vi "Initialize Sweep Waveform.vi"(8 "error in (no error)":errorcluster, 11 "Instrument.DAQ in":refnum<class "Instrument.DAQ.lvclass">) -> (0 "error out":errorcluster, 2 "Waveforms":waveform(dbl)[](array[waveform]), 3 "Instrument.DAQ out":refnum<class "Instrument.DAQ.lvclass">)   [LabVIEW 2019, in "Instrument.Lockin.lvlib" / "Instrument.DAQ.lvclass"]
uses:
  Instrument.DAQ.lvclass
  Instrument.DAQ.lvclass/Instrument.DAQ.ctl
  <vilib>/Utility/error.llb/Error Cluster From Error Code.vi
  <vilib>/ErrorRing/Error Ring.xnode
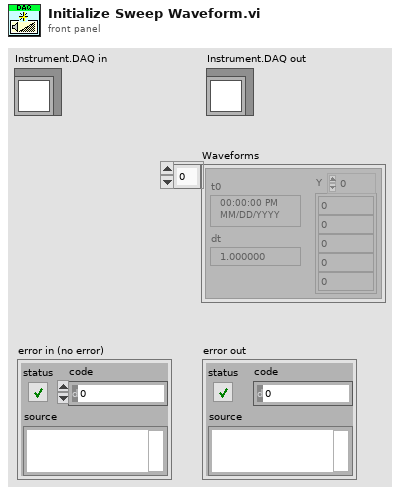
[diagram p1: front panel]
types:
  T1 = typedef "Instrument.Lockin.lvlib/Instrument.DAQ.lvclass/AO.Channel--Cluster--Array.ctl" = T2[]
  T2 = typedef "Instrument.Lockin.lvlib/Instrument.DAQ.lvclass/AO.Channel--Cluster.ctl" = cluster{"Enable?":bool, "Channel":i32, "Amplitude":dbl, "Offset":dbl, "Frequency":dbl, "Phase":dbl, "Function":T3, "Sweeping?":bool}
  T3 = typedef "Instrument.Lockin.lvlib/Instrument.DAQ.lvclass/AO.Channel.Function--Enum.ctl" = enum16{"Sine", "Triangle", "Square"}
  T4 = typedef "Instrument.Lockin.lvlib/Instrument.DAQ.lvclass/Sweep.Channel--Cluster--Array.ctl" = T5[]
  T5 = typedef "Instrument.Lockin.lvlib/Instrument.DAQ.lvclass/Sweep.Channel--Cluster.ctl" = cluster{"Enable?":bool, "Channel":u16, "Start":dbl, "End":dbl, "Pattern":T6, "Table":dbl[]}
  T6 = typedef "Instrument.Lockin.lvlib/Instrument.DAQ.lvclass/Sweep.Pattern--Enum.ctl" = enum16{"Ramp /", "Ramp /\\", "Smooth Ramp _/", "Smooth Ramp _/\\_", "Table"}
  T7 = typedef "Instrument.Lockin.lvlib/Instrument.DAQ.lvclass/DAQ.Sampling.Sampling--Cluster.ctl" = cluster{"Fs":dbl, "#s":i32}
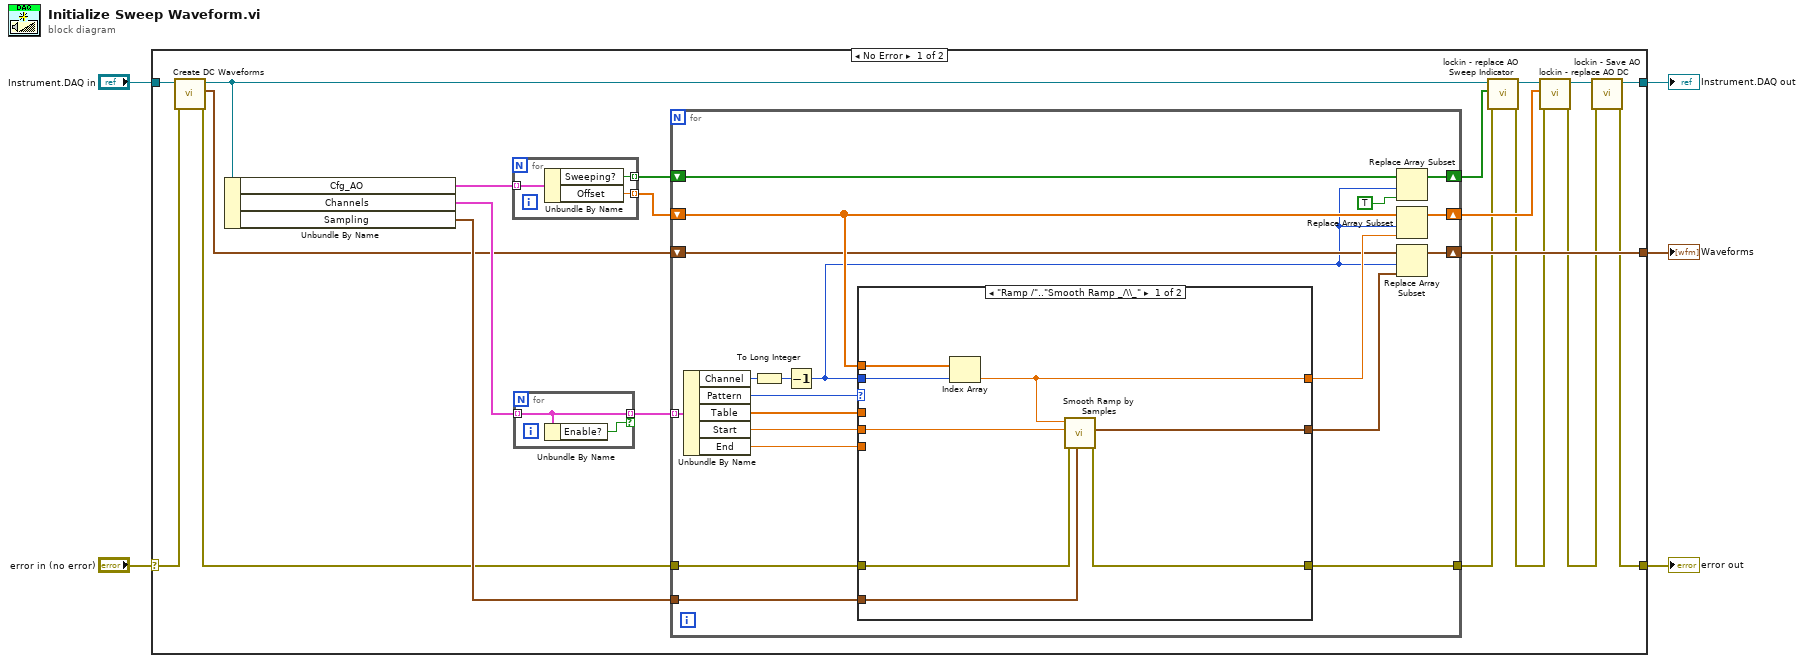
[diagram p0: block diagram]
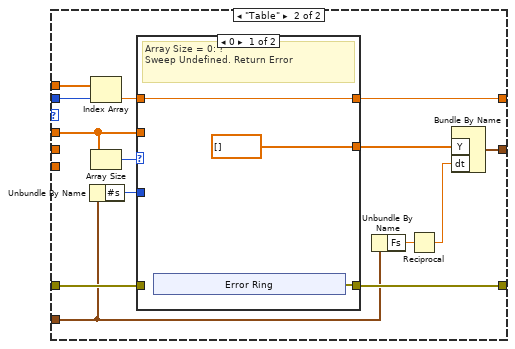
[diagram p2: hidden frame]
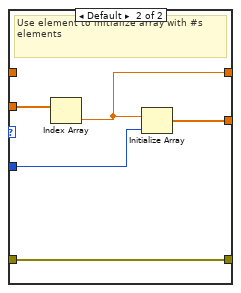
[diagram p3: hidden frame]
diagram:
  n1 = case shown="No Error" "error in (no error)" {
    selector: "error in (no error)" -> [w18 w88]
    tunnel: "Instrument.DAQ in" -> [w19 w87]
    tunnel: [w8 w88] -> w2
    tunnel: [w7 w87] -> w1
    tunnel: [w20 _] -> w3
    frame No Error {
      n2 = call "Create DC Waveforms.vi"("error in (no error)"=w18, "Instrument.DAQ in"=w19) -> ("Error out"=w17:errorcluster, "Waveforms []"=w16:waveform(dbl)[], "Instrument.DAQ out"=w6:refnum<class "Instrument.DAQ.lvclass">)  [unwired: 7 in]
      n3 = Unbundle By Name(w6) -> ("Cfg_AO"=w22:T1, "Channels"=w21:T4, "Sampling"=w26:T7)
      n4 = for {
        tunnel: [w29] -> w24 mode=indexing
        tunnel: [w28] -> w23 mode=indexing
        tunnel: w22 -> [w27] mode=indexing
        n5 = Unbundle By Name(w27) -> ("Sweeping?"=w28:bool, "Offset"=w29:dbl)
      }
      n6 = for {
        tunnel: w21 -> [w86] mode=indexing
        tunnel: [w86] -> w25 mode=indexing if=w85
        n7 = Unbundle By Name(w86) -> ("Enable?"=w85:bool)
      }
      n8 = for {
        tunnel: w17 -> [w49]
        tunnel: w25 -> [w44] mode=indexing
        tunnel: w26 -> [w43]
        tunnel: [w42] -> w11
        shift-right: [w38] -> w13
        shift-left: w23 -> [w40]
        shift-right: [w39] -> w12
        shift-left: w24 -> [w37]
        shift-right: [w34] -> w20
        shift-left: w16 -> [w33]
        n9 = Unbundle By Name(w44) -> ("Channel"=w36:u16, "Pattern"=w47:T6, "Table"=w48:dbl[], "Start"=w46:dbl, "End"=w45:dbl)
        n10 = To Long Integer(number=w36) -> (32bit integer=w30:i32)
        n11 = Decrement(x=w30) -> (x-1=w32:i32)
        n12 = case shown="\"Ramp /\"..\"Smooth Ramp _/\\\\_\"" w47 {
          tunnel: w45 -> [_ _]
          tunnel: w46 -> [w52 _]
          tunnel: [w50 w70] -> w42
          tunnel: w49 -> [w57 w71]
          tunnel: w43 -> [w53 w66]
          tunnel: w48 -> [_ w69]
          tunnel: [w56 w64] -> w31
          tunnel: w37 -> [w55 w60]
          tunnel: w32 -> [w54 w59]
          tunnel: [w51 w61] -> w35
          frame "Ramp /".."Smooth Ramp _/\\_" {
            n13 = Index Array(array=w55, index=w54) -> (element=w51:dbl)
            n14 = call "Smooth Ramp by Samples.vi"("sampling"=w53, "error in (no error)"=w57, "End"=w52, "Start"=w51) -> ("Error out"=w50:errorcluster, "output waveform"=w56:waveform(dbl))  [unwired: 6 in]
          }
          frame "Table" {
            n15 = Unbundle By Name(w66) -> ("#s"=w67:i32)
            n16 = Index Array(array=w60, index=w59) -> (element=w58:dbl)
            n17 = Array Size(array=w69) -> (size(s)=w68:i32)
            n18 = case shown="0" w68 {
              tunnel: w71 -> [_ w81]
              tunnel: [w73 w81] -> w70
              tunnel: [dbl[] [] ("Y") w83] -> w62
              tunnel: w67 -> [_ w82]
              tunnel: w69 -> [_ w84]
              tunnel: [w72 w80] -> w61
              tunnel: w58 -> [w72 _]
              frame 0 {
                # "Array Size = 0: ?\nSweep Undefined. Return Error"
                n19 = xnode "Error Ring"() -> ("error out"=w73:errorcluster)
              }
              frame Default {
                # "Use element to initialize array with #s elements"
                n20 = Index Array(array=w84) -> (element=w80:dbl)  [unwired: 1 in]
                n21 = Initialize Array(w80, w82) -> (w83:dbl[])
              }
            }
            n22 = Unbundle By Name(w66) -> ("Fs"=w65:dbl)
            n23 = Reciprocal(x=w65) -> (1/x=w63:dbl)
            n24 = Bundle By Name("Y"=w62, "dt"=w63) -> (w64:waveform(dbl))  [unwired: 1 in]
          }
        }
        n25 = Replace Array Subset(array=w40, new element=TRUE ("new element/subarray"), index=w32) -> (w38:bool[])
        n26 = Replace Array Subset(array=w37, new element=w35, index=w32) -> (w39:dbl[])
        n27 = Replace Array Subset(array=w33, new element=w31, index=w32) -> (w34:waveform(dbl)[])
      }
      n28 = call "lockin - replace AO Sweep Indicator.vi"("error in (no error)"=w11, "Channels: AO.Sweeping?"=w13, "Instrument.DAQ"=w6) -> ("error out"=w10:errorcluster, "Instrument.DAQout"=w14:refnum<class "Instrument.DAQ.lvclass">)  [unwired: 7 in]
      n29 = call "lockin - replace AO DC.vi"("error in (no error)"=w10, "AO.DC (V)"=w12, "Instrument.DAQ"=w14) -> ("error out"=w9:errorcluster, "Instrument.DAQ out"=w15:refnum<class "Instrument.DAQ.lvclass">)  [unwired: 7 in]
      n30 = call "lockin - Save AO.vi"("error in (no error)"=w9, "Instrument.DAQ"=w15) -> ("error out"=w8:errorcluster, "Instrument.DAQ out"=w7:refnum<class "Instrument.DAQ.lvclass">)  [unwired: 8 in]
    }
    frame Error {
    }
  }
  "Instrument.DAQ out" <- w1
  "error out" <- w2
  "Waveforms" <- w3
